vi "Panel.vi"(11 "BP Summary in":refnum<class "BP Summary.lvclass">) -> ()   [LabVIEW 2020, in "BP Summary.lvclass"]
uses:
  BP Summary.lvclass
  C:/Program Files (x86)/National Instruments/LabVIEW 2020/vi.lib/IlluminatedG/IG OOPanel/OOPanel/Panel/Panel.lvclass
  C:/Program Files (x86)/National Instruments/LabVIEW 2020/vi.lib/IlluminatedG/IG OOPanel/OOPanel/ArrayPanel/ArrayPanel.lvclass
  BP Summary.lvclass/BP Summary.ctl
  App/Blueprint Qty.ctl
  Blueprint/Blueprint.lvclass
  BP Item/BP Item.lvclass
  <vilib>/IlluminatedG/IG OOPanel/OOPanel/Panel/Panel.lvclass
  Workstation/Workstation.lvclass
  <vilib>/IlluminatedG/IG OOPanel/OOPanel/ArrayManager/ArrayManager.lvclass
  <vilib>/IlluminatedG/IG OOPanel/OOPanel/ArrayPanel/ArrayPanel.lvclass
  App/App.lvclass
panel:
  in  "BD":bool
  out "Assembled At":string
  in  "Show Components":bool
  in  "Qty":dbl min=0.0 step=1.0
  out "Craft Time":dbl
  out "Name":string
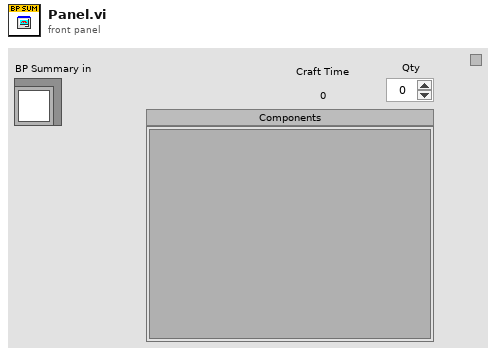
[diagram p1: front panel]
types:
  T1 = typedef "Item.lvclass/Ingredient.ctl" = cluster{"Item":refnum<class "Item.lvclass">, "Qty":dbl}
  T2 = typedef "Item.lvclass/Craft Station.ctl" = cluster{"Station":refnum<class "Workstation.lvclass">, "Craft Time":dbl, "Qty Made":dbl}
  T3 = typedef "App.lvclass/Blueprint Qty.ctl" = cluster{"Blueprint":refnum<class "Blueprint.lvclass">, "Qty":dbl}
  T4 = typedef "BP Summary.lvclass/Ref Data.ctl" = cluster{"Show Components":bool}
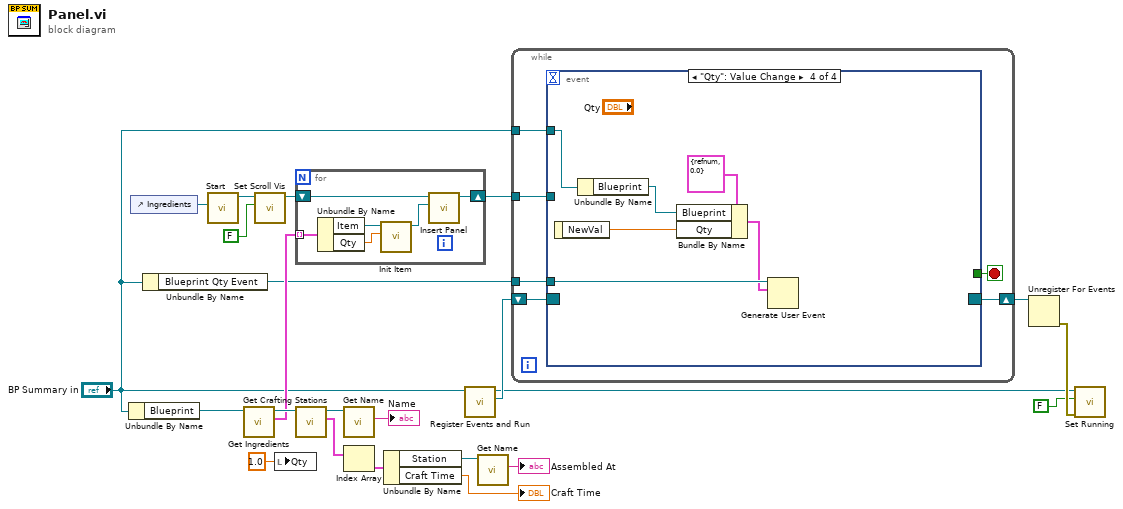
[diagram p0: block diagram]
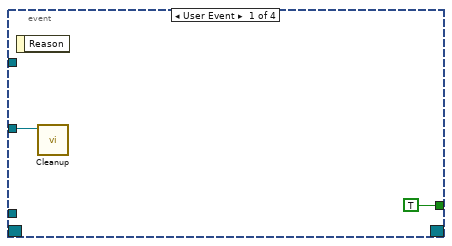
[diagram p2: hidden frame]
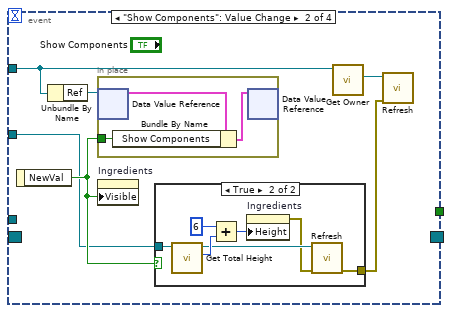
[diagram p3: hidden frame]
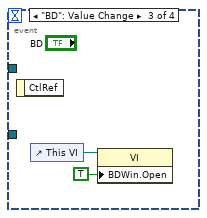
[diagram p5: hidden frame]
diagram:
  n1 = Unbundle By Name("BP Summary in") -> ("Blueprint"=w10:refnum<class "Blueprint.lvclass">)
  n2 = control-ref of="Ingredients"() -> (w7:refnum<vi>)
  n3 = Unbundle By Name("BP Summary in") -> ("Blueprint Qty Event"=w1:refnum<user-event>)
  n4 = call <vilib>:"Start.vi"("Container"=w7) -> ("ArrayManager out"=w5:refnum<class "ArrayManager.lvclass">)  [unwired: 9 in, 1 out]
  n5 = call-dynamic "Get Ingredients.vi"("Blueprint in"=w10) -> ("Ingredients"=w8:T1[], "Blueprint out"=w9:refnum<class "Blueprint.lvclass">)  [unwired: 8 in, 1 out]
  n6 = call <vilib>:"Set Scroll Vis.vi"("Scroll Visible"=FALSE, "ArrayManager in"=w5) -> ("ArrayManager out"=w4:refnum<class "ArrayManager.lvclass">)  [unwired: 8 in, 1 out]
  n7 = local write "Qty"(1.0 ("Qty")) -> ()
  n8 = for {
    tunnel: w8 -> [w29] mode=indexing
    shift-right: [w24] -> w6
    shift-left: w4 -> [w26]
    n9 = Unbundle By Name(w29) -> ("Item"=w28:refnum<class "Item.lvclass">, "Qty"=w27:dbl)
    n10 = call "Init Item.vi"("Qty"=w27, "Item"=w28) -> ("BP Item out"=w25:refnum<class "BP Item.lvclass">)  [unwired: 8 in, 1 out]
    n11 = call <vilib>:"Insert Panel.vi"("Panel/Type"=w25, "PanelArray in"=w26) -> ("PanelArray out"=w24:refnum<class "ArrayManager.lvclass">)  [unwired: 7 in, 2 out]
  }
  n12 = call-dynamic "Get Crafting Stations.vi"("Blueprint in"=w9) -> ("Stations"=w17:T2[], "Blueprint out"=w11:refnum<class "Blueprint.lvclass">)  [unwired: 8 in, 1 out]
  n13 = call-dynamic "Get Name.vi"("Blueprint in"=w11) -> ("Name"=→"Name":string)  [unwired: 8 in, 2 out]
  n14 = Index Array(array=w17) -> (element=w16:T2)  [unwired: 1 in]
  n15 = Unbundle By Name(w16) -> ("Station"=w15:refnum<class "Workstation.lvclass">, "Craft Time"=→"Craft Time":dbl)
  n16 = call <vilib>:"Register Events and Run.vi"("Panel in"="BP Summary in") -> ("Panel Event Reg"=w23:refnum<event-registration>, "Panel out"=w19:refnum<class "BP Summary.lvclass">)  [unwired: 8 in, 1 out]
  n17 = call "Get Name.vi"("Workstation in"=w15) -> ("Name"=→"Assembled At":string)  [unwired: 8 in, 2 out]
  n18 = while {
    shift-right: [w34] -> w22
    shift-left: w23 -> [w35]
    tunnel: "BP Summary in" -> [w32]
    tunnel: w6 -> [w31]
    tunnel: w1 -> [w30]
    stop <- w33 stop-if-true
    n19 = event shown="[3] \"Qty\": Value Change" {
      selector: w35 -> [_ _ _ _]
      dyn-events: [_ _ _ _] -> w34
      timeout: _ -> [_ _ _ _]
      tunnel: [TRUE _ _ _] -> w33
      tunnel: w32 -> [_ w38 _ w57]
      tunnel: w31 -> [w36 w41 _ _]
      tunnel: w30 -> [_ _ _ w61]
      event User Event {
        n20 = event-data() -> ()  [unwired: 1 in, 1 out]
        n21 = call <vilib>:"Cleanup.vi"("PanelArray in"=w36) -> ()  [unwired: 10 in, 1 out]
      }
      event "Show Components": Value Change {
        n22 = event-data() -> ("NewVal"=w42:bool)  [unwired: 1 in]
        n23 = Unbundle By Name(w38) -> ("Ref"=w43:refnum<data-value>)
        n24 = in-place {
          in-place-border: w42 -> [w51]
          n25 = in-place-dvr #1(w43) -> (w53:T4)  [unwired: 1 out]
          n26 = Bundle By Name(cluster=w53, "Show Components"=w51) -> (w52:T4)
          n27 = in-place-dvr #1(w52) -> ()  [unwired: 2 out]
        }
        n28 = property on="Ingredients" class="SubPnl"("Visible"=w42) -> ()  [unwired: 2 in, 2 out]
        n29 = case shown="True" w42 {
          tunnel: w41 -> [_ w50]
          tunnel: [_ w44] -> w40
          frame False {
          }
          frame True {
            n30 = call <vilib>:"Get Total Height.vi"("ArrayManager in"=w50) -> ("Total Height"=w49:u32, "ArrayManager out"=w46:refnum<class "ArrayManager.lvclass">)  [unwired: 8 in, 1 out]
            n31 = Add(x=u32 6, y=w49) -> (x+y=w48:u32)
            n32 = property on="Ingredients" class="SubPnl"("Height"=w48) -> (error out=w45:errorcluster)  [unwired: 2 in, 1 out]
            n33 = call <vilib>:"Refresh.vi"("error in (no error)"=w45, "ArrayManager in"=w46) -> ("error out"=w44:errorcluster)  [unwired: 8 in, 1 out]
          }
        }
        n34 = call <vilib>:"Get Owner.vi"("ArrayPanel in"=w38) -> ("Owner"=w39:refnum<class "ArrayManager.lvclass">)  [unwired: 8 in, 2 out]
        n35 = call <vilib>:"Refresh.vi"("error in (no error)"=w40, "ArrayManager in"=w39) -> ()  [unwired: 8 in, 2 out]
      }
      event "BD": Value Change {
        n36 = event-data() -> ()  [unwired: 1 in, 1 out]
        n37 = control-ref of="This VI"() -> (w55:refnum<vi>)
        n38 = property class="VI"(reference=w55, "BDWin.Open"=TRUE ("Block Diagram Window:Open")) -> ()  [unwired: 1 in, 2 out]
      }
      event "Qty": Value Change {
        n39 = event-data() -> ("NewVal"=w58:dbl)  [unwired: 1 in]
        n40 = Unbundle By Name(w57) -> ("Blueprint"=w56:refnum<class "Blueprint.lvclass">)
        n41 = Bundle By Name(cluster=T3 {"Blueprint"=refnum, "Qty"=0.0} ("event data"), "Blueprint"=w56, "Qty"=w58) -> (w59:T3)
        n42 = Generate User Event(user event=w61, event data cluster=w59) -> ()  [unwired: 2 in, 2 out]
      }
    }
  }
  n43 = Unregister For Events(event registration refnum=w22) -> (error out=w21:errorcluster)  [unwired: 1 in]
  n44 = call <vilib>:"Set Running.vi"("error in (no error)"=w21, "Running"=FALSE, "Panel in"=w19) -> ()  [unwired: 7 in, 2 out]
